vi "PWM_Motor_IR.vi"(0 "Sensorwert":dbl, 1 "Geschwindigkeit multiplikator":dbl(knob) scale=0.0..1.0) -> (6 "PWM Motor":dbl=0.3)   [LabVIEW 2016]
doc: "Geschwindigkeitsregelung anhand IR Sensor vorne\n05.04.17_Tloe"
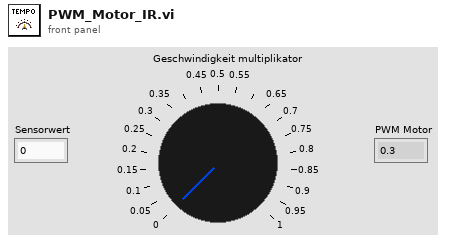
[diagram p1: front panel]
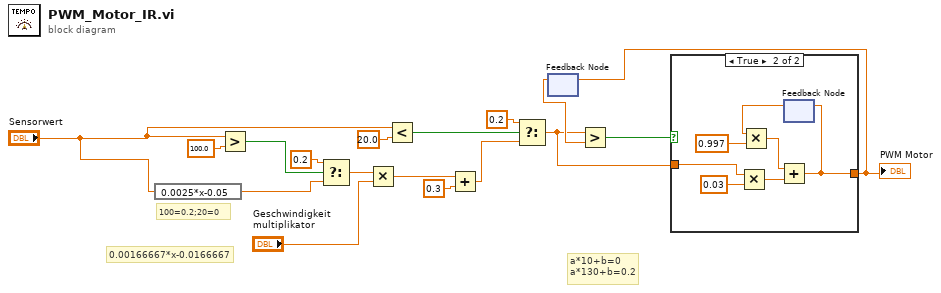
[diagram p0: block diagram]
diagram:
  # "100=0.2;20=0"
  # "0.00166667*x-0.0166667"
  # "a*10+b=0 \na*130+b=0.2"
  n1 = expression code="0.0025*x-0.05"("Sensorwert") -> (w10:dbl)
  n2 = Greater?(x="Sensorwert", y=100.0) -> (0:w16:bool)
  n3 = Select(t=0.2, s=w16, f=w10) -> (s? t:f=w13:dbl)
  n4 = Multiply(x=w13, y="Geschwindigkeit multiplikator") -> (x*y=w14:dbl)
  n5 = Less?(x="Sensorwert", y=20.0) -> (x < y?=w8:bool)
  n6 = Add(x=w14, y=0.3) -> (x+y=w9:dbl)
  n7 = Select(t=0.2, s=w8, f=w9) -> (s? t:f=w3:dbl)
  n8 = feedback #1() -> (w4:dbl)  [unwired: 1 in]
  n9 = Greater?(x=w3, y=w4) -> (0:w5:bool)
  n10 = case shown="True" w5 {
    tunnel: w3 -> [w18 w20]
    tunnel: [w18 w19] -> w2
    frame False {
    }
    frame True {
      n11 = Multiply(x=w20, y=0.03) -> (x*y=w22:dbl)
      n12 = feedback #2() -> (w25:dbl)  [unwired: 1 in]
      n13 = Multiply(x=w25, y=0.997) -> (x*y=w24:dbl)
      n14 = Add(x=w24, y=w22) -> (x+y=w19:dbl)
      n15 = feedback-in #2(w19) -> ()
    }
  }
  "PWM Motor" <- w2
  n16 = feedback-in #1(w2) -> ()
